vi "Select Node Class by type.vi"(11 "Value":string) -> (3 "Node out":refnum<class "Node.lvclass">)   [LabVIEW 2025]
uses:
  Classes/Node/Node.lvclass
  Classes/Node/Array/Array Control/Array Control.lvclass
  C:/Users/mrjak/Documents/GitHub/LVGPT/LabVIEW/VIs/Classes/Node/Node.lvclass
  Classes/Node/GrowableFunction/GrowableFunction.lvclass
  Classes/Node/Control/Bool Control/Bool Control.lvclass
  Classes/Node/Constant/Boolean Constant/Boolean Constant.lvclass
  Classes/MultiDiagramStructure/MultiDiagramStructure.lvclass
  Classes/ProeprtyNode/PropertyNode.lvclass
  Classes/Node/Control/Numeric Control/Numeric Control.lvclass
  Classes/Node/Constant/Numeric Constant/Numeric Constant.lvclass
  Classes/Node/Constant/String Constant/String Constant.lvclass
  Classes/Node/Control/String Control/String Control.lvclass
  Classes/Node/Function/Function.lvclass
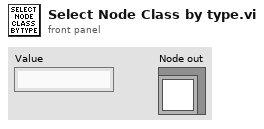
[diagram p1: front panel]
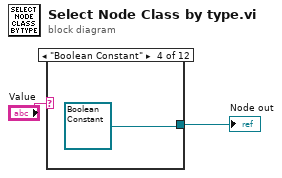
[diagram p0: block diagram]
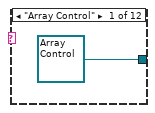
[diagram p2: hidden frame]
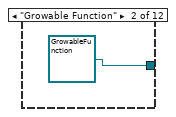
[diagram p3: hidden frame]
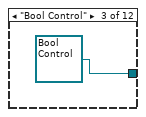
[diagram p4: hidden frame]
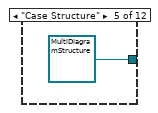
[diagram p5: hidden frame]
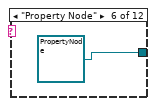
[diagram p6: hidden frame]
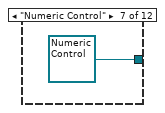
[diagram p7: hidden frame]
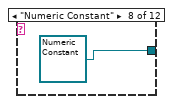
[diagram p8: hidden frame]
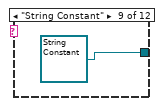
[diagram p9: hidden frame]
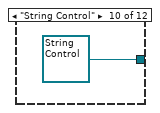
[diagram p10: hidden frame]
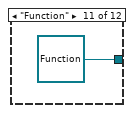
[diagram p11: hidden frame]
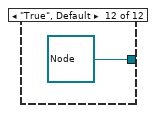
[diagram p12: hidden frame]
diagram:
  n1 = case shown="\"Boolean Constant\"" "Value" {
    tunnel: [refnum<class "Array Control.lvclass"> refnum ("Array Control.lvclass") refnum<class "GrowableFunction.lvclass"> refnum ("GrowableFunction.lvclass") refnum<class "Bool Control.lvclass"> refnum ("Bool Control.lvclass") refnum<class "Boolean Constant.lvclass"> refnum ("Boolean Constant.lvclass") refnum<class "MultiDiagramStructure.lvclass"> refnum ("MultiDiagramStructure.lvclass") refnum<class "PropertyNode.lvclass"> refnum ("PropertyNode.lvclass") refnum<class "Numeric Control.lvclass"> refnum ("Numeric Control.lvclass") refnum<class "Numeric Constant.lvclass"> refnum ("Numeric Constant.lvclass") refnum<class "String Constant.lvclass"> refnum ("String Constant.lvclass") refnum<class "String Control.lvclass"> refnum ("String Control.lvclass") refnum<class "Function.lvclass"> refnum ("Function.lvclass") refnum<class "Node.lvclass"> refnum ("Node.lvclass")] -> w1
    frame "Array Control" {
    }
    frame "Growable Function" {
    }
    frame "Bool Control" {
    }
    frame "Boolean Constant" {
    }
    frame "Case Structure" {
    }
    frame "Property Node" {
    }
    frame "Numeric Control" {
    }
    frame "Numeric Constant" {
    }
    frame "String Constant" {
    }
    frame "String Control" {
    }
    frame "Function" {
    }
    frame "True", Default {
    }
  }
  "Node out" <- w1
